vi "Read App.vi"(8 "error in (no error)":errorcluster, 11 "Application Test In":refnum<class "Application Dev Test.lvclass">) -> (0 "error out":errorcluster, 2 "App out":refnum<class "Application.lvclass">, 3 "Application Test Out":refnum<class "Application Dev Test.lvclass">)   [LabVIEW 2020, in "Application Dev Test.lvclass"]
uses:
  Application Dev Test.lvclass
  source/Framework/Application/Application.lvclass
  C:/Git/astemes-triarc-framework/source/Framework Test/Base Class Test/Base Test.lvclass
  source/Framework Test Suite/Base Class Test/Base Test.lvclass/Base Test.ctl
  source/Framework/Base/Base.lvclass
  Application Dev Test.lvclass/Application Dev Test.ctl
  source/Framework Test Suite/Base Class Test/Base Test.lvclass
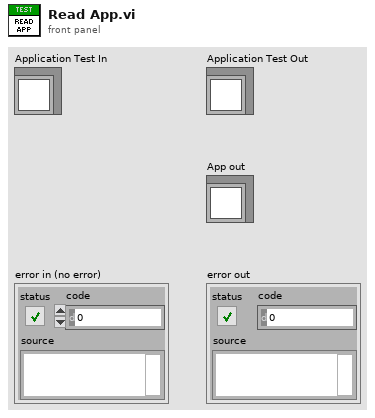
[diagram p1: front panel]
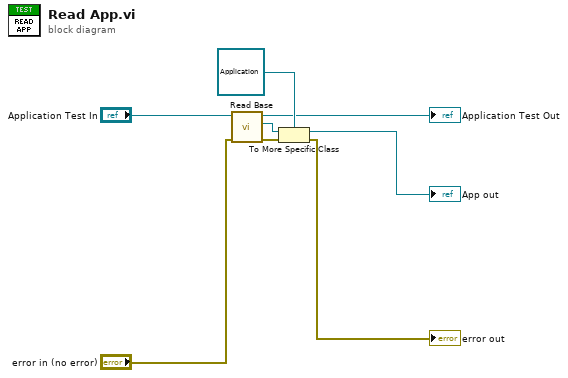
[diagram p0: block diagram]
diagram:
  n1 = call "Read Base.vi"("error in (no error)"="error in (no error)", "Base Class Test In"="Application Test In") -> ("error out"=w4:errorcluster, "Base.lvclass"=w5:refnum<class "Base.lvclass">, "Base Class Test Out"=→"Application Test Out":refnum<class "Application Dev Test.lvclass">)  [unwired: 7 in]
  n2 = To More Specific Class(target class=refnum<class "Application.lvclass"> refnum ("Rig in"), reference=w5, error in=w4) -> (specific class reference=→"App out":refnum<class "Application.lvclass">, error out=→"error out":errorcluster)
